vi "SP - get subpanel ref.vi"(8 "error in (no error)":errorcluster, 11 "subpanel":string) -> (0 "error out":errorcluster, 2 "subpanel found ?":bool, 3 "subpanel ref":refnum<vi>)   [LabVIEW 2020, in "ui-testing.lvlib"]
uses:
  ui-testing.lvlib
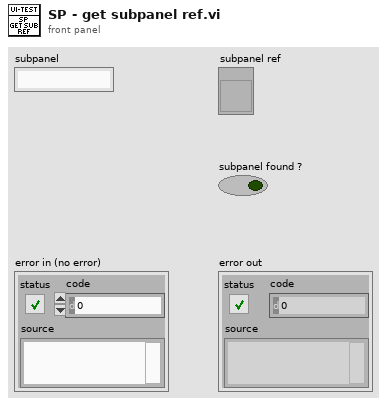
[diagram p1: front panel]
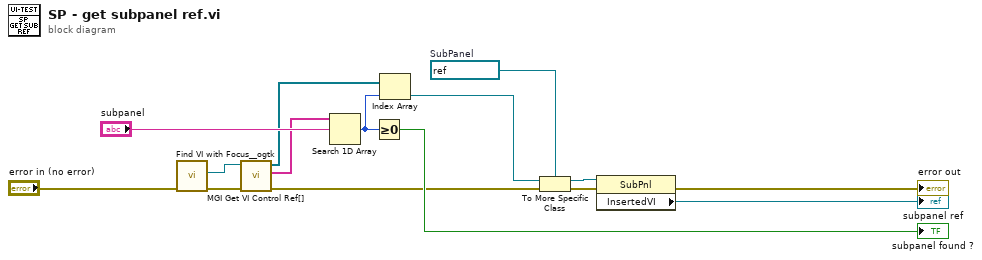
[diagram p0: block diagram]
diagram:
  w10 = refnum<vi> refnum  # SubPanel
  n1 = call <userlib>:"Find VI with Focus__ogtk.vi"("error in"="error in (no error)") -> ("error out"=w8:errorcluster, "VI with Focus"=w5:refnum<vi>)  [unwired: 6 in, 3 out]
  n2 = call <userlib>:"MGI Get VI Control Ref[].vi"("error in"=w8, "VI (Caller)"=w5) -> ("error out"=w9:errorcluster, "Control Label Chain[i]"=w3:string[], "Control[i]"=w2:refnum<vi>[])  [unwired: 6 in, 1 out]
  n3 = Search 1D Array(1D array=w3, element="subpanel") -> (index of element=w4:i32)  [unwired: 1 in]
  n4 = Greater Or Equal To 0?(x=w4) -> (x >= 0?=→"subpanel found ?":bool)
  n5 = Index Array(array=w2, index=w4) -> (element=w6:refnum<vi>)
  n6 = To More Specific Class(target class=w10, reference=w6, error in=w9) -> (specific class reference=w11:refnum<vi>, error out=w12:errorcluster)
  n7 = property class="SubPnl"(reference=w11, error in=w12) -> (error out=→"error out":errorcluster, "InsertedVI"=→"subpanel ref":refnum<vi>)  [unwired: 1 out]
